vi "Max Power Point Tracker.vi"(6 "Scan settings":T1={"J-V scan"=FALSE, "J-t scan"=FALSE, "Min (V)"=0.0, "Max (V)"=0.0, "Step (V)"=0.0, "Measurement delay (ms)"=10.0, "1st scan FB-SC"=FALSE, "Inverted structure"=FALSE, "Stabilisation time (s)"=0.0, "Stabilisation mode"=enum."V", "Stabilisation value (V or A) "=0.0, "Step time (s)"=0.0, "Integration time"=enum."Fast", "Repeat each scan 10 times"=FALSE, "Dark J-V only"=FALSE, "Light and dark measurements"=FALSE, "Only measure in dark for best pixel"=FALSE, "All measurements under light"=FALSE}, 7 "Cell details cluster":T2={"Cell Position"=16, "Cell Label"="", "Pixel to measure"=0, "Area (cm^2)"=0.126, "Variable"="", "Variable value"="", "Scan settings in queue"=0, "Light or dark"=""} {"Pixel to measure" items=["All", "1", "2", "3", "4", "5", "6", "7", "8"]}, 10 "Experiment Title":string, 11 "User Name":string) -> (3 "Jt Curve":cluster{"Y":dbl[], "Y":dbl[]}[](graph) caption="JV Curve")   [LabVIEW 2011]
uses:
  <instrlib>/keithley_24xx/Keithley 24XX/Keithley 24XX.lvlib
  <instrlib>/keithley_24xx/Keithley 24XX/Public/Data/Read (Single Point).vi
panel:
  in  "MaxPow Stabilisation time (s)":dbl
  in  "Initial voltage":dbl
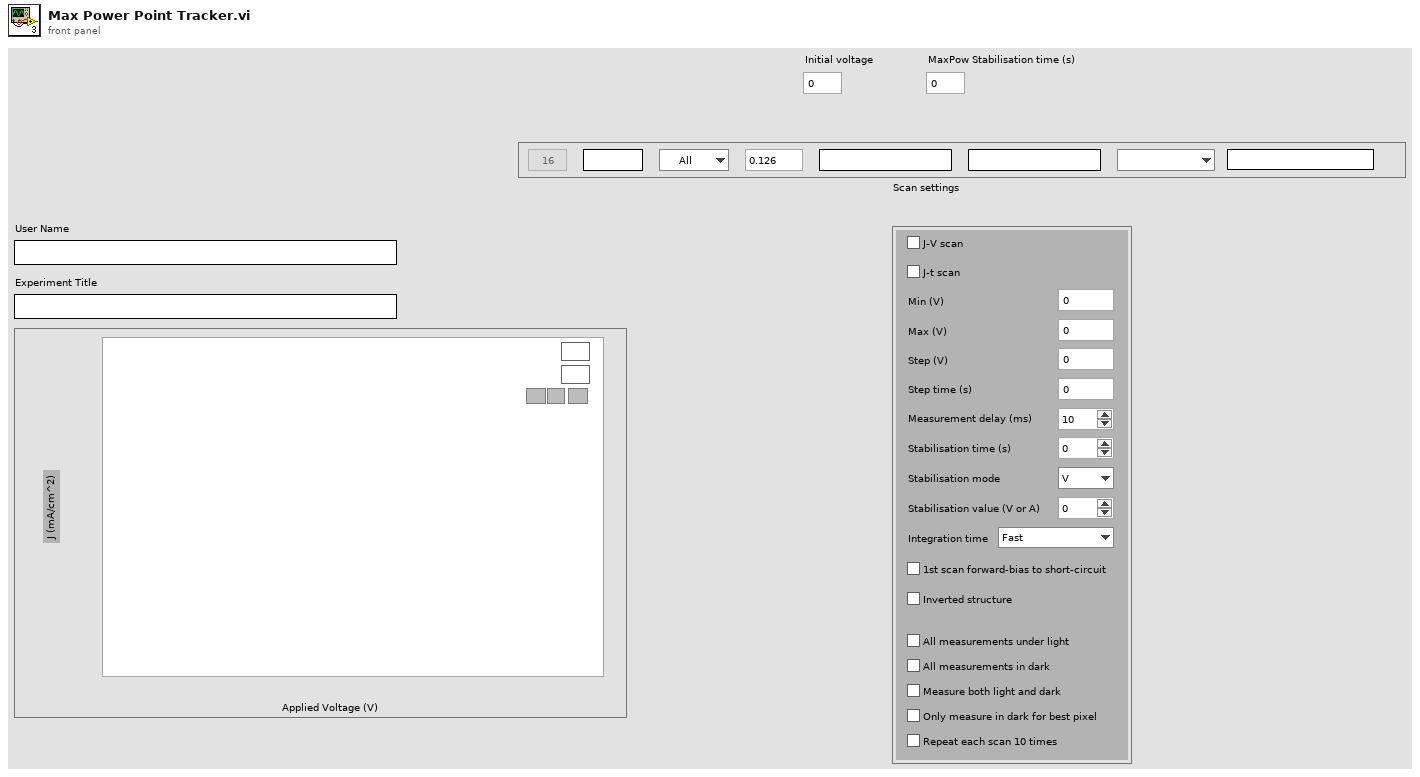
[diagram p1: front panel]
types:
  T1 = cluster{"J-V scan":bool, "J-t scan":bool, "Min (V)":dbl, "Max (V)":dbl, "Step (V)":dbl, "Measurement delay (ms)":dbl, "1st scan FB-SC":bool, "Inverted structure":bool, "Stabilisation time (s)":dbl, "Stabilisation mode":enum16{"V", "I"}, "Stabilisation value (V or A) ":dbl, "Step time (s)":dbl, "Integration time":enum16{"Fast", "Normal", "High Accuracy"}, "Repeat each scan 10 times":bool, "Dark J-V only":bool, "Light and dark measurements":bool, "Only measure in dark for best pixel":bool, "All measurements under light":bool}
  T2 = cluster{"Cell Position":i32, "Cell Label":string, "Pixel to measure":u16, "Area (cm^2)":dbl, "Variable":string, "Variable value":string, "Scan settings in queue":u16, "Light or dark":string}
  T3 = typedef "imagedata.ctl" = cluster{"image type":i32, "image depth":i32, "image":u8[], "mask":u8[], "colors":u32[], "Rectangle":cluster{"left":i16, "top":i16, "right":i16, "bottom":i16}}
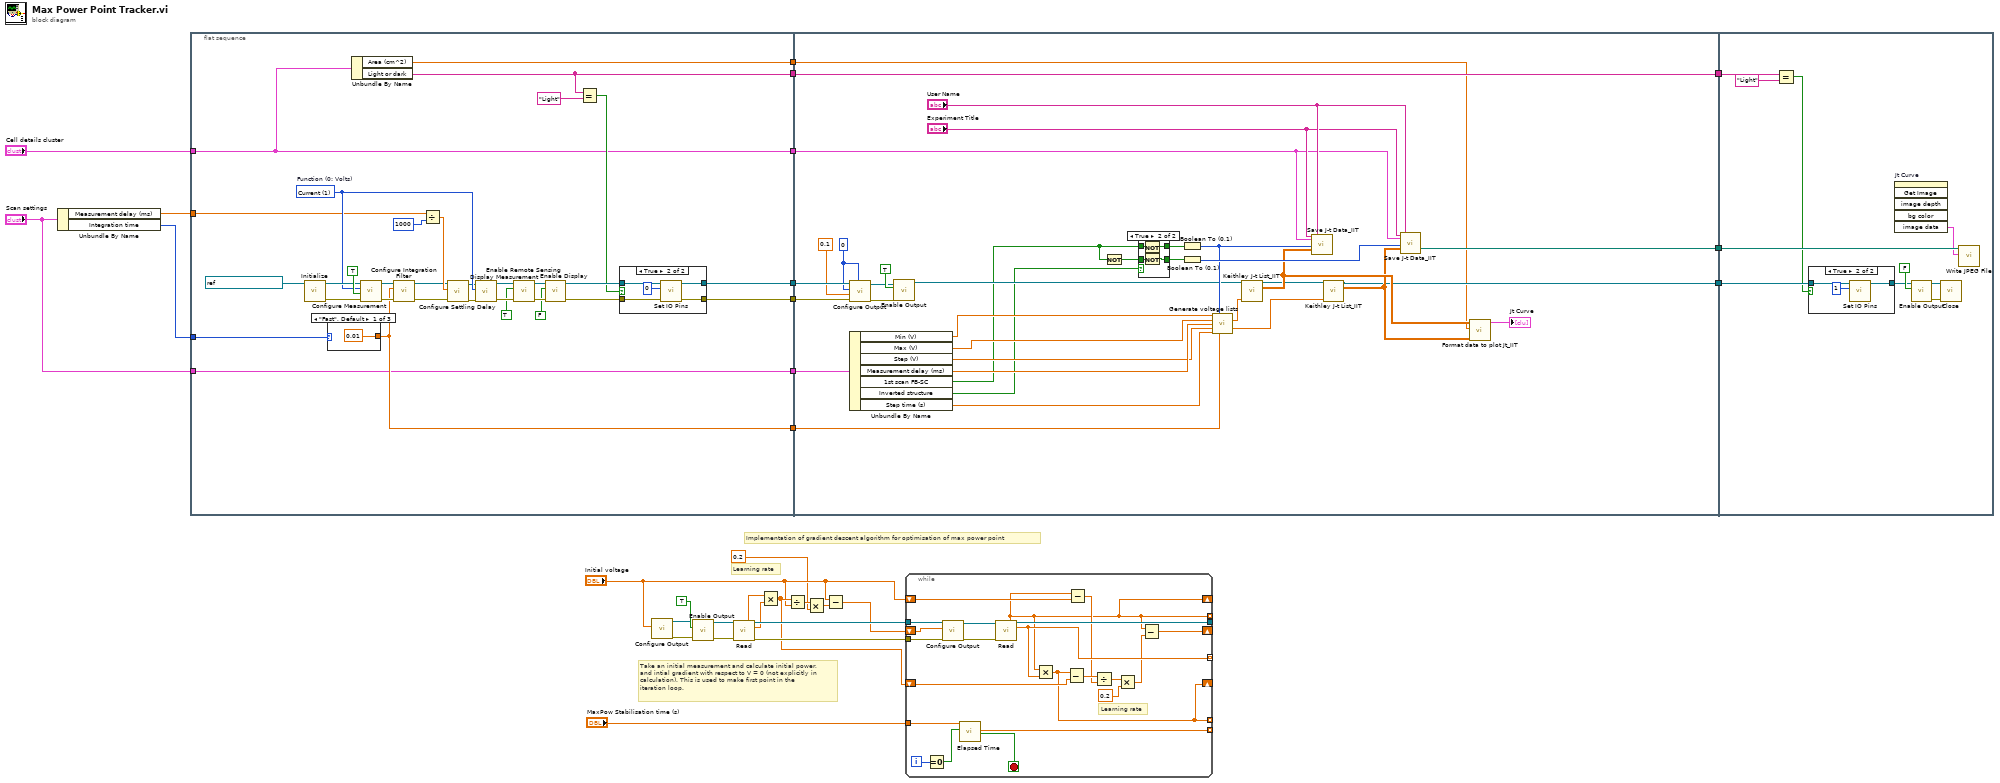
[diagram p0: block diagram]
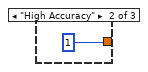
[diagram p3: hidden frame]
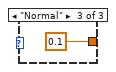
[diagram p4: hidden frame]
diagram:
  # "Learning rate"
  # "Take an initial measurement and calculate initial power,\nand intial gradient with respect to V = 0 (not explicitly in\ncalculation). This is used to make first point in the\niteration loop."
  # "Implementation of gradient descent algorithm for optimisation of max power point"
  n1 = Unbundle By Name("Scan settings") -> ("Measurement delay (ms)"=w24:dbl, "Integration time"=w25:enum16{"Fast", "Normal", "High Accuracy"})
  n2 = flat-sequence {
    tunnel: [w35] -> w29
    tunnel: [w36] -> w30
    tunnel: [w43] -> w28
    tunnel: w25 -> [w42]
    tunnel: w24 -> [w41]
    tunnel: [w33] -> w23
    tunnel: "Cell details cluster" -> [w33]
    tunnel: [w40] -> w21
    tunnel: "Scan settings" -> [w40]
    tunnel: [w32] -> w18
    tunnel: [w31] -> w17
    tunnel: [w88] -> w27
    tunnel: [w104] -> w26
    tunnel: w30 -> [w101]
    tunnel: w29 -> [w100]
    tunnel: w28 -> [w95]
    tunnel: w23 -> [w73]
    tunnel: w21 -> [w85]
    tunnel: [w75] -> w19
    tunnel: w18 -> [w75]
    tunnel: w17 -> [w74]
    tunnel: w27 -> [w117]
    tunnel: w26 -> [w120]
    tunnel: w19 -> [w114]
    frame #0 {
      w51 = u16 1 items=["Volts", "Current", "Resistance"]  # Function (0: Volts)
      n3 = call <instrlib>:"Initialize.vi"("VISA resource name"=refnum<visa-resource-name> "GPIB0::24::INSTR") -> ("error out"=w55:errorcluster, "VISA resource name out"=w56:refnum<visa-resource-name>)  [unwired: 4 in, 5 out]
      n4 = case shown="\"Fast\", Default" w42 {
        tunnel: [0.01 1 0.1] -> w43
        frame "Fast", Default {
        }
        frame "High Accuracy" {
        }
        frame "Normal" {
        }
      }
      n5 = Unbundle By Name(w33) -> ("Area (cm^2)"=w31:dbl, "Light or dark"=w32:string)
      n6 = call <instrlib>:"Configure Measurement.vi"("error in (no error)"=w55, "Enable Auto Range (T:Enable)"=TRUE, "Function (0: Volts)"=w51, "VISA resource name"=w56) -> ("error out"=w58:errorcluster, "VISA resource name out"=w57:refnum<visa-resource-name>)  [unwired: 6 in]
      n7 = call <instrlib>:"Configure Integration Filter.vi"("error in (no error)"=w58, "Measurement Speed (1 PLC)"=w43, "VISA resource name"=w57) -> ("error out"=w44:errorcluster, "VISA resource name out"=w47:refnum<visa-resource-name>)  [unwired: 7 in]
      n8 = Divide(x=w41, y=1000) -> (x/y=w49:dbl)
      n9 = call <instrlib>:"Configure Settling Delay.vi"("error in (no error)"=w44, "Manual Settling Delay (0 sec)"=w49, "VISA resource name"=w47) -> ("error out"=w45:errorcluster, "VISA resource name out"=w46:refnum<visa-resource-name>)  [unwired: 7 in]
      n10 = call <instrlib>:"Display Measurement.vi"("error in (no error)"=w45, "Displayed Measurement (0: Voltage)"=w51, "VISA resource name"=w46) -> ("error out"=w60:errorcluster, "VISA resource name out"=w59:refnum<visa-resource-name>)  [unwired: 7 in]
      n11 = call <instrlib>:"Enable Remote Sensing.vi"("error in (no error)"=w60, "Enable Remote Sensing (T: Enable)"=TRUE ("Enable Output (T: Enable)"), "VISA resource name"=w59) -> ("error out"=w53:errorcluster, "VISA resource name out"=w54:refnum<visa-resource-name>)  [unwired: 7 in]
      n12 = call <instrlib>:"Enable Display.vi"("error in (no error)"=w53, "Enable Display (T: Enable)"=FALSE ("Enable Output (T: Enable)"), "VISA resource name"=w54) -> ("error out"=w37:errorcluster, "VISA resource name out"=w38:refnum<visa-resource-name>)  [unwired: 7 in]
      n13 = Equal?(x=w32, y="Light") -> (x = y?=w34:bool)
      n14 = case shown="True" w34 {
        tunnel: w38 -> [w64 w68]
        tunnel: w37 -> [w63 w67]
        tunnel: [w64 w66] -> w36
        tunnel: [w63 w65] -> w35
        frame False {
        }
        frame True {
          n15 = call <instrlib>:"Set IO Pins.vi"("error in (no error)"=w67, "Output Pattern (0)"=0, "VISA resource name"=w68) -> ("error out"=w65:errorcluster, "VISA resource name out"=w66:refnum<visa-resource-name>)  [unwired: 7 in]
        }
      }
    }
    frame #1 {
      w97 = 0
      n16 = call <instrlib>:"Configure Output.vi"("Source Mode  (0: Voltage)"=w97, "error in (no error)"=w100, "Compliance  Level (0.1)"=0.1, "Output Level (0)"=w97, "VISA resource name"=w101) -> ("error out"=w98:errorcluster, "VISA resource name out"=w99:refnum<visa-resource-name>)  [unwired: 5 in]
      n17 = Unbundle By Name(w85) -> ("Min (V)"=w84:dbl, "Max (V)"=w83:dbl, "Step (V)"=w81:dbl, "Measurement delay (ms)"=w82:dbl, "1st scan FB-SC"=w79:bool, "Inverted structure"=w78:bool, "Step time (s)"=w80:dbl)
      n18 = call <instrlib>:"Enable Output.vi"("error in (no error)"=w98, "Enable Output (T: Enable)"=TRUE ("Output (Off)"), "VISA resource name"=w99) -> ("VISA resource name out"=w94:refnum<visa-resource-name>)  [unwired: 7 in, 1 out]
      n19 = Not(x=w79) -> (.not. x?=w105:bool)
      n20 = case shown="True" w78 {
        tunnel: [w109 w113] -> w107
        tunnel: [w108 w112] -> w106
        tunnel: w105 -> [w108 w111]
        tunnel: w79 -> [w109 w110]
        frame False {
        }
        frame True {
          n21 = Not(x=w110) -> (.not. x?=w113:bool)
          n22 = Not(x=w111) -> (.not. x?=w112:bool)
        }
      }
      n23 = Boolean To (0,1)(Boolean=w107) -> (0, 1=w96:i16)
      n24 = Boolean To (0,1)(Boolean=w106) -> (0, 1=w102:i16)
      n25 = call "Generate voltage lists.vi"("MinVoltage"=w84, "Initial sweep direction"=w96, "Max Voltage"=w83, "Measurement Delay (ms)"=w82, "V step"=w81, "t step"=w80, "NPLC"=w95) -> ("Voltage Forward List"=w93:dbl[], "Voltage Reverse List"=w90:dbl[])  [unwired: 7 in]
      n26 = call "Keithley J-t List_IIT.vi"("VISA resource name in"=w94, "Voltage List"=w93) -> ("VISA resource name out"=w91:refnum<visa-resource-name>, "Data Array"=w92:dbl[][])  [unwired: 11 in, 1 out]
      n27 = call "Save J-t Data_IIT.vi"("Experiment Indicator"="Experiment Title", "Cell details cluster"=w73, "Scan direction"=w96, "Data Array"=w92, "Username"="User Name") -> ()  [unwired: 13 in, 2 out]
      n28 = call "Keithley J-t List_IIT.vi"("VISA resource name in"=w91, "Voltage List"=w90) -> ("VISA resource name out"=w88:refnum<visa-resource-name>, "Data Array"=w89:dbl[][])  [unwired: 11 in, 1 out]
      n29 = call "Save J-t Data_IIT.vi"("Experiment Indicator"="Experiment Title", "Cell details cluster"=w73, "Scan direction"=w102, "Data Array"=w89, "Username"="User Name") -> ("File path for JV image"=w104:path)  [unwired: 13 in, 1 out]
      n30 = call "Format data to plot Jt_IIT.vi"("Data Array 2"=w89, "Device Area (cm^2)"=w74, "Data Array"=w92) -> ("JV Curve"=→"Jt Curve":cluster{"Y":dbl[], "Y":dbl[]}[])  [unwired: 8 in]
    }
    frame #2 {
      n31 = Equal?(x=w114, y="Light") -> (x = y?=w115:bool)
      n32 = case shown="True" w115 {
        tunnel: w117 -> [w124 w126]
        tunnel: [w124 w125] -> w116
        frame False {
        }
        frame True {
          n33 = call <instrlib>:"Set IO Pins.vi"("Output Pattern (0)"=1, "VISA resource name"=w126) -> ("VISA resource name out"=w125:refnum<visa-resource-name>)  [unwired: 8 in, 1 out]
        }
      }
      n34 = invoke on="Jt Curve" class="XYGraph (strict)" method="Get Image"() -> ("image data"=w119:T3)  [unwired: 6 in, 5 out]
      n35 = call <instrlib>:"Enable Output.vi"("Enable Output (T: Enable)"=FALSE ("Output (Off)"), "VISA resource name"=w116) -> ("error out"=w122:errorcluster, "VISA resource name out"=w123:refnum<visa-resource-name>)  [unwired: 8 in]
      n36 = call <instrlib>:"Close.vi"("error in (no error)"=w122, "VISA resource name"=w123) -> ()  [unwired: 9 in, 1 out]
      n37 = call <vilib>:"Write JPEG File.vi"("image data"=w119, "path to JPEG file"=w120) -> ()  [unwired: 8 in, 2 out]
    }
  }
  n38 = call <instrlib>:"Configure Output.vi"("Output Level (0)"="Initial voltage") -> ("error out"=w14:errorcluster, "VISA resource name out"=w15:refnum<visa-resource-name>)  [unwired: 9 in]
  n39 = call <instrlib>:"Enable Output.vi"("error in (no error)"=w14, "Enable Output (T: Enable)"=TRUE ("Output (Off)"), "VISA resource name"=w15) -> ("error out"=w12:errorcluster, "VISA resource name out"=w13:refnum<visa-resource-name>)  [unwired: 7 in]
  n40 = call-poly <instrlib>:"Read.vi"("VISA resource name"=w13, "error in (no error)"=w12) -> ("Voltage"=w9:sgl, "VISA resource name out"=w11:refnum<visa-resource-name>, "Current"=w8:sgl, "error out"=w10:errorcluster)  [unwired: 7 in, 3 out]
  n41 = Multiply(x=w9, y=w8) -> (x*y=w3:sgl)
  n42 = Divide(x=w3, y="Initial voltage") -> (x/y=w7:dbl)
  n43 = Multiply(x=w7, y=0.2) -> (x*y=w6:dbl)
  n44 = Subtract(x="Initial voltage", y=w6) -> (x-y=w5:dbl)
  n45 = while {
    tunnel: w11 -> [w143]
    tunnel: w10 -> [w142]
    tunnel: [w149] -> _
    tunnel: [w147] -> _ mode=indexing
    tunnel: [w138] -> _ mode=indexing
    tunnel: "MaxPow Stabilisation time (s)" -> [w144]
    shift-right: [w130] -> _
    shift-left: w5 -> [w139]
    shift-right: [w129] -> _
    shift-left: w3 -> [w137]
    shift-right: [w128] -> _
    shift-left: "Initial voltage" -> [w135]
    tunnel: [w129] -> _ mode=indexing
    tunnel: [w128] -> _ mode=indexing
    i -> [w146]
    stop <- w148 stop-if-true
    # "Learning rate"
    n46 = Equal To 0?(x=w146) -> (x = 0?=w145:bool)
    n47 = call <instrlib>:"Configure Output.vi"("error in (no error)"=w142, "Output Level (0)"=w139, "VISA resource name"=w143) -> ("error out"=w140:errorcluster, "VISA resource name out"=w141:refnum<visa-resource-name>)  [unwired: 7 in]
    n48 = call "Elapsed Time"("Time Target (s)"=w144, "Reset"=w145) -> ("Elapsed Time (s)"=w147:dbl, "Time has Elapsed"=w148:bool)  [unwired: 10 in, 6 out]
    n49 = call-poly <instrlib>:"Read.vi"("VISA resource name"=w141, "error in (no error)"=w140) -> ("Voltage"=w128:sgl, "VISA resource name out"=w149:refnum<visa-resource-name>, "Current"=w138:sgl)  [unwired: 7 in, 4 out]
    n50 = Multiply(x=w128, y=w138) -> (x*y=w129:sgl)
    n51 = Subtract(x=w129, y=w137) -> (x-y=w136:sgl)
    n52 = Subtract(x=w128, y=w135) -> (x-y=w134:dbl)
    n53 = Divide(x=w136, y=w134) -> (x/y=w133:dbl)
    n54 = Multiply(x=w133, y=0.2) -> (x*y=w131:dbl)
    n55 = Subtract(x=w128, y=w131) -> (x-y=w130:dbl)
  }
